vi "acquire sequence to disk.vi"(0 "Image Size":T4={"H Bin"=1, "V Bin"=1, "Left"=1, "Top"=1, "Right"=512, "Bottom"=512} {"Top" min=4 max=2048 step=4; "Left" min=4 max=2048 step=4; "V Bin" min=1 max=2048 step=4; "H Bin" min=1 max=2048 step=4}, 1 "Display?":bool=TRUE, 2 "State In":T5 {"Height" format="%.2f"; "Width" format="%.2f"}, 3 "Frames per acquisition file":u32, 4 "Sequence files handle":T3, 6 "Description Info":string, 7 "Pressing stop automatically runs finish?":bool=TRUE, 9 "Display Window Title":string="Acquired Image", 10 "Operation":enum16{"Start", "Continue", "Finish"}(ring), 11 "Display Window Number":i32, 12 "Number of frames to acquire":i32) -> (15 "Done?":bool, 16 "State Out":T5 {"Height" format="%.2f"; "Width" format="%.2f"}, 18 "Sequence files handle out":T3, 19 "error out":errorcluster)   [LabVIEW 2015]
doc: "Acquires a video sequence into the acquisition RAID directory using the camera handle and buffers already set up (e.g., by ixon acquisition setup.vi). \n\nUse as a sub-vi:\n\nSTARTING: If Start (T)/Continue (F) is True, starts the acquisition from frame 1 and \"State In\" is ignored. If false, continues an earlier acquistision that was temporarily interrupted, using information in \"State In\". \n\nSTOPPING: Program always stops acquisition by calling Camera Stop before it exits. Stop is temporary if Number of frames to acquire is > 0 and the number of frames acquired exceeds that value. In that case, State Out is set so that acquisition can be resumed later. In contrast, if acquisition is stopped by pressing \"Stop\", by an error, or by setting STOP=true as input, the acquisition is over permanently. In that case,the vi writes the header file and frees the acquisition buffers."
uses:
  Glimpse core/Video acquisition state.ctl
  <vilib>/vision/Image Controls.llb/IMAQ Image.ctl
  Glimpse core/Seq file v 1/Offset table.ctl
  Glimpse core/Seq file v 1/Offset.ctl
  Glimpse core/Seq file v 1/file number.ctl
  ixon camera/image size.ctl
  Glimpse core/Sequence files handle.ctt
  h-nu-ixon/Emission filters.ctl
  h-nu-ixon/Laser type.ctt
  ixon1024/HAL camera parameters important.ctt
  ixon1024/ixon readout settings.ctl
  ixon1024/andor acquisition mode.ctl
  Glimpse core/Header2 file data.ctl
  Glimpse core/GLIMPSE Globals.vi
  h-nu-ixon/stage globals.vi
  h-nu shutters/hardware status globals.vi
  fluid handling/Flow cell controller globals.vi
  h-nu-ixon/Microscope ID global.vi
  ixon1024/HAL Camera specifications globals.vi
  Microscope software version global.vi
panel:
  in  "Laser\n(to get strings only)":T1
  in  "Emission filter\n(to get strings only)":T2
  out "Channel switch overhead (ms)":u32
  out "Sequence files directory path":path
  in  "stop":bool
  out "Frame interval (ms)":i16
  out "TTB element zero":u32
  out "Time of 1st frame":dbl
  out "Frames Acquired":u32(slide) scale=0.0..10000.0
  # "Parameters for non-interactive use"
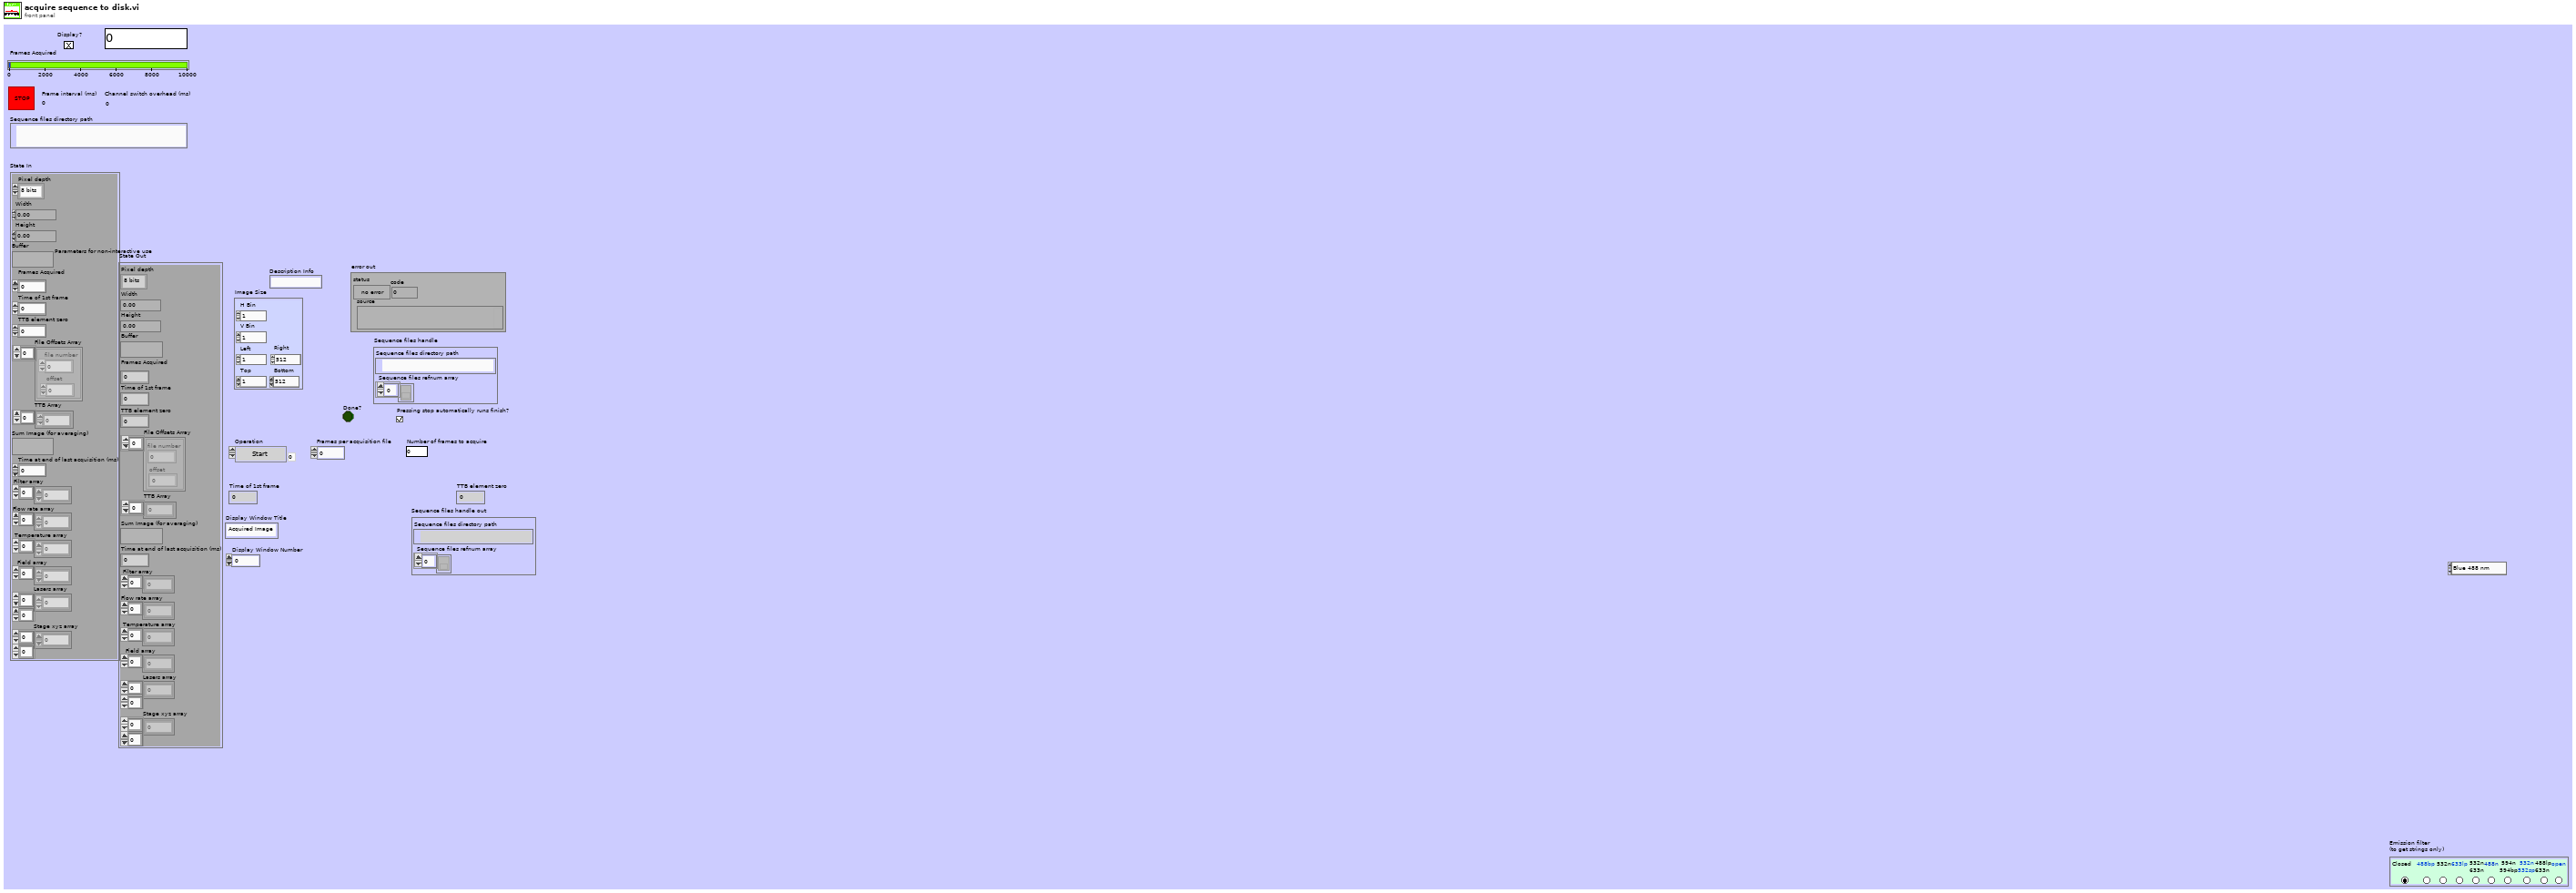
[diagram p1: front panel]
types:
  T1 = typedef "Laser type.ctt" = enum16{"Blue 488 nm", "Green 532 nm", "Orange 594 nm", "Red 633 nm", "IR 780"}
  T2 = typedef "Emission filters.ctl" = enum32{" Closed ", "488bp ", "532n", "633lp ", "532n\n633n", "488n", "594n\n594bp", "532n\n532sp", "488lp\n633n", "open"}
  T3 = typedef "Sequence files handle.ctt" = cluster{"Sequence files directory path":path, "Sequence files refnum array":refnum<file>[]}
  T4 = typedef "image size.ctl" = cluster{"H Bin":i32, "V Bin":i32, "Left":i32, "Top":i32, "Right":i32, "Bottom":i32}
  T5 = typedef "Video acquisition state.ctl" = cluster{"Pixel depth":enum32{"8 bits", "16 bits", "Float", "Complex", "RGB Chunky", "Compressed"}, "Width":dbl, "Height":dbl, "Buffer":T6, "Frames Acquired":u32, "Time of 1st frame":dbl, "TTB element zero":u32, "File Offsets Array":T7, "TTB Array":u32[], "Sum Image (for averaging)":T6, "Time at end of last acquisition (ms)":u32, "Filter array":u16[], "Flow rate array":dbl[], "Temperature array":dbl[], "Field array":u16[], "Lasers array":u16[][], "Stage xyz array":dbl[][]}
  T6 = typedef "IMAQ Image.ctl" = refnum<image>
  T7 = typedef "Offset table.ctl" = cluster{"offset":T8, "file number":T9}[]
  T8 = typedef "Offset.ctl" = i32
  T9 = typedef "file number.ctl" = u8
  T10 = enum32{"8 bits", "16 bits", "Float", "Complex", "RGB Chunky", "Compressed"}
  T11 = typedef "HAL camera parameters important.ctt" = cluster{"Exposure Time (sec)":sgl, "EM CCD Gain":u16, "Readout Settings":T12, "Image Size":cluster{"H Bin":i32, "V Bin":i32, "Left":i32, "Top":i32, "Right":i32, "Bottom":i32}}
  T12 = typedef "ixon readout settings.ctl" = cluster{"Acquisition Mode":T13, "Pixel Rate":enum16{"EM CCD 10 Mhz 14 bits", "EM CCD 5 Mhz 14 bits", "EM CCD 3 Mhz 14 bits", "EM CCD 1 Mhz 16 bits", "Standard CCD 3 Mhz 14 bits", "Standard CCD 1 Mhz 16 bits"}, "High Capacity?":bool, "V Shift Speed (us/row)":enum16{"0.9 (not reccommended)", "1.7  (not reccommended)", "3.3  (not reccommended)", "6.5", "12.9"}, "V Shift Amplitude":enum16{"normal", "+1", "+2", "+3", "+4"}, "Preamp Gain":enum16{"1.0", "2.4", "5.0"}, "Trigger Mode":u32, "Baseline offset":i16, "Baseline clamp":bool}
  T13 = typedef "andor acquisition mode.ctl" = enum16{"(do not use)", "Single Scan", "Accumulate", "Kinetics", "Fast Kinetics", "Kinetics Run till Abort", "Frame Transfer", "Frame Transfer Run till Abort", "(do not use) ", "Time Delayed Integration"}
  T14 = typedef "shutters status.ctl" = cluster{"Laser":T1, "Status":bool}[]
  T15 = typedef "Header2 file data.ctl" = cluster{"Camera":string, "Microscope":string, "Microscope software version":string, "Laser names":string[], "Filter names":string[], "Lasers array":u16[][], "Filter array":u16[], "Flow rate array":dbl[], "Temperature array":dbl[], "Field array":u16[], "Is header2 info present?":bool, "Description Info":string, "Stage xyz array":dbl[][]}
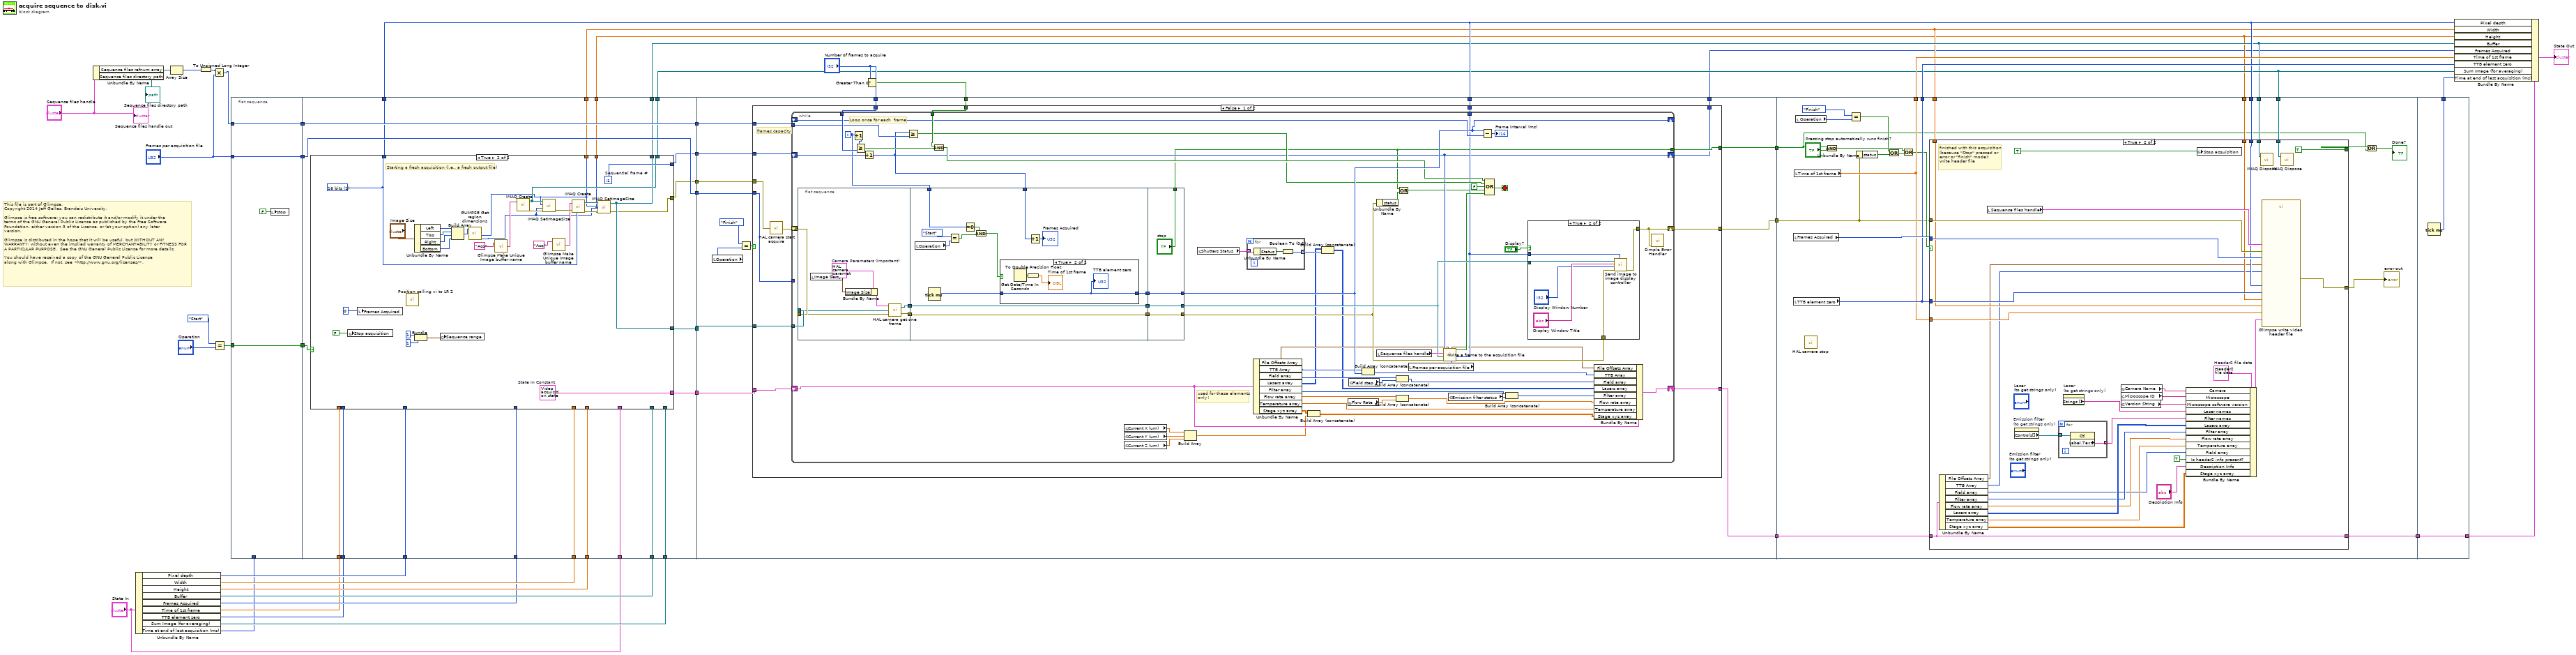
[diagram p0: block diagram]
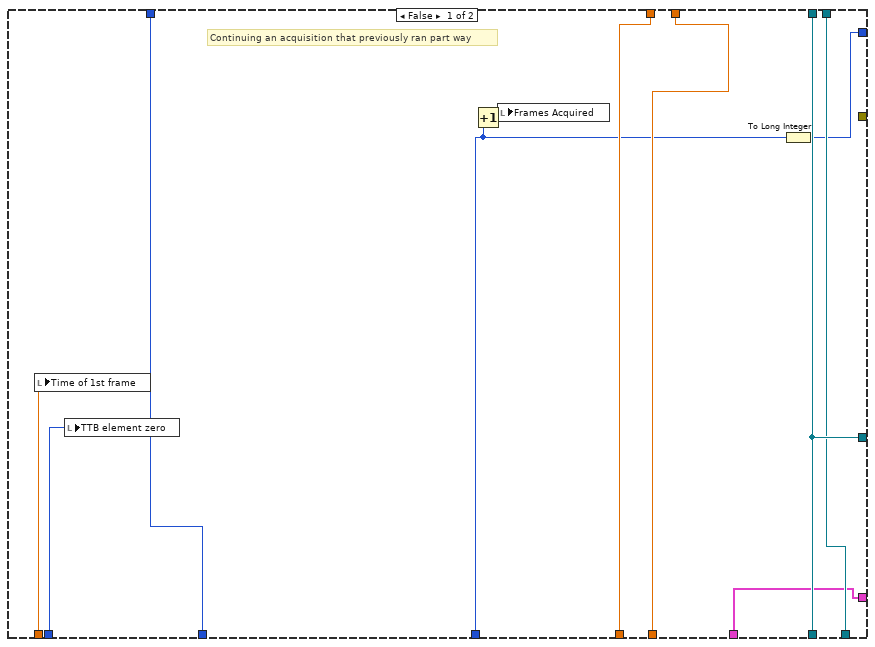
[diagram p2: hidden frame]
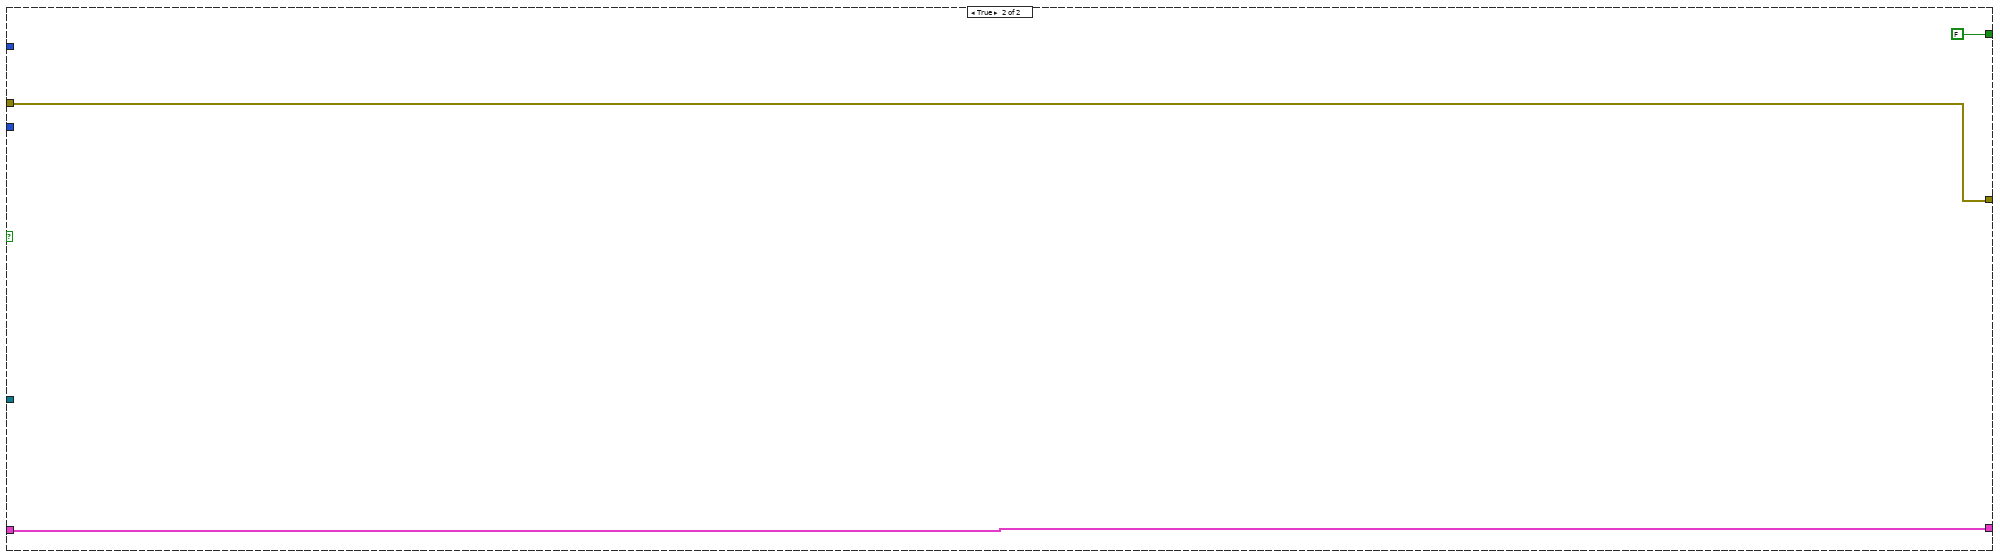
[diagram p5: hidden frame]
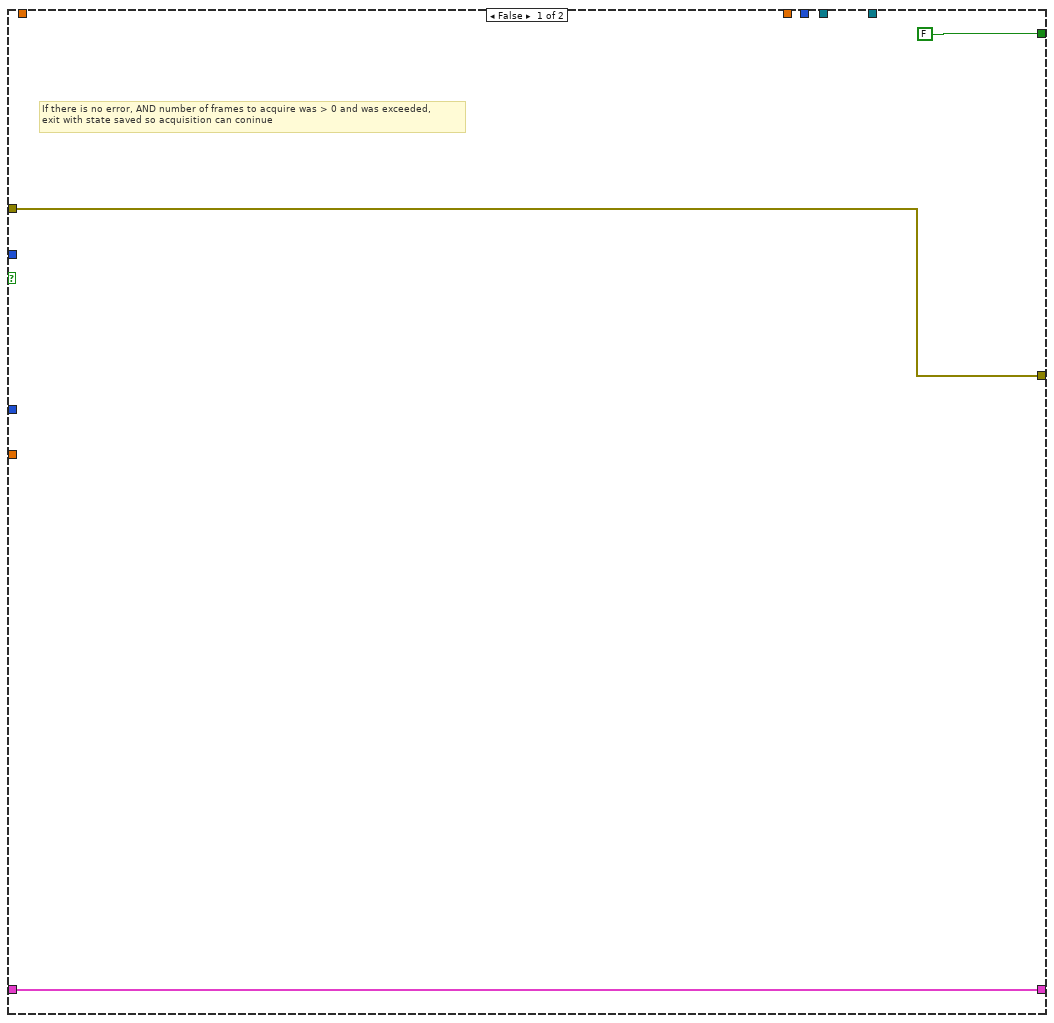
[diagram p6: hidden frame]
diagram:
  # "This file is part of Glimpse. \nCopyright 2014 Jeff Gelles, Brandeis University.    \n\nGlimpse is free software: you can redistribute it and/or modify it under the \nterms of the GNU General Public License as published by the Free Software \nFoundation, either version 3 of the License, or (at your option) any later \nversion.\n\nGlimpse is distributed in the hope that it will be useful, but WITHOUT ANY \nWARRANTY; without even the implied warranty of MERCHANTABILITY or FITNESS FOR \nA PARTICULAR PURPOSE.  See the GNU General Public License for more details.\n\nYou should have received a copy of the GNU General Public License\nalong with Glimpse.  If not, see <http://www.gnu.org/licenses/>."
  n1 = Unbundle By Name("Sequence files handle") -> ("Sequence files refnum array"=w9:refnum<file>[], "Sequence files directory path"=→"Sequence files directory path":path)
  n2 = Unbundle By Name("State In") -> ("Pixel depth"=w36:T10, "Width"=w35:dbl, "Height"=w34:dbl, "Buffer"=w33:T6, "Frames Acquired"=w32:u32, "Time of 1st frame"=w30:dbl, "TTB element zero"=w29:u32, "Sum Image (for averaging)"=w25:T6, "Time at end of last acquisition (ms)"=w6:u32)
  n3 = Array Size(array=w9) -> (size(s)=w26:i32)
  n4 = To Unsigned Long Integer(number=w26) -> (unsigned 32bit integer=w45:u32)
  n5 = Multiply(x=w45, y="Frames per acquisition file") -> (x*y=w46:u32)
  n6 = Equal?(x=enum16{"Start", "Continue", "Finish"}."Start", y="Operation") -> (x = y?=w19:bool)
  n7 = flat-sequence {
    tunnel: w19 -> [w51]
    tunnel: "Frames per acquisition file" -> [w52]
    tunnel: w46 -> [w53]
    tunnel: [w53] -> w13
    tunnel: [w52] -> w12
    tunnel: [w51] -> w11
    tunnel: w6 -> [w47]
    tunnel: [w73] -> w41
    tunnel: [w72] -> w40
    tunnel: [w71] -> w39
    tunnel: [w70] -> w38
    tunnel: [w69] -> w22
    tunnel: [w68] -> w16
    tunnel: [w67] -> w15
    tunnel: [w66] -> w20
    tunnel: w36 -> [w65]
    tunnel: w35 -> [w64]
    tunnel: w34 -> [w56]
    tunnel: w33 -> [w63]
    tunnel: w32 -> [w62]
    tunnel: [w61] -> w31
    tunnel: w30 -> [w60]
    tunnel: w29 -> [w59]
    tunnel: w25 -> [w58]
    tunnel: [w57] -> w21
    tunnel: w13 -> [w73]
    tunnel: w12 -> [w72]
    tunnel: w11 -> [w74]
    tunnel: "State In" -> [w55]
    tunnel: [w54] -> w4
    tunnel: w41 -> [w128]
    tunnel: w40 -> [w127]
    tunnel: [w122] -> w42
    tunnel: w39 -> [w116]
    tunnel: w38 -> [w126]
    tunnel: w31 -> [w125]
    tunnel: "Number of frames to acquire" -> [w124]
    tunnel: w23 -> [w123]
    tunnel: w22 -> [w121]
    tunnel: [w120] -> w17
    tunnel: [w115] -> w14
    tunnel: w4 -> [w114]
    tunnel: [w113] -> w3
    tunnel: w42 -> [w245]
    tunnel: [w264] -> w28
    tunnel: [w263] -> w27
    tunnel: w15 -> [w262]
    tunnel: w16 -> [w261]
    tunnel: w22 -> [w260]
    tunnel: w21 -> [w257]
    tunnel: w20 -> [w256]
    tunnel: w17 -> [w246]
    tunnel: w3 -> [w244]
    tunnel: [w243] -> w2
    tunnel: [w304] -> w7
    tunnel: [w303] -> w1
    tunnel: w2 -> [w303]
    frame #0 {
      n8 = Tick Count (ms)() -> (millisecond timer value=w48:u32)
      n9 = Subtract(x=w48, y=w47) -> (x-y=→"Channel switch overhead (ms)":u32)
      n10 = local write "stop"(FALSE ("stop")) -> ()
    }
    frame #1 {
      n11 = case shown="True" w74 {
        tunnel: [_ w101] -> w71
        tunnel: [w77 w105] -> w70
        tunnel: [w81 w95] -> w69
        tunnel: [w85 w88] -> w68
        tunnel: [w84 w87] -> w67
        tunnel: [w82 w104] -> w66
        tunnel: w65 -> [w81 _]
        tunnel: w64 -> [w85 _]
        tunnel: w56 -> [w84 _]
        tunnel: w63 -> [w82 _]
        tunnel: w62 -> [w83 _]
        tunnel: [w82 w104] -> w61
        tunnel: w60 -> [w80 _]
        tunnel: w59 -> [w79 _]
        tunnel: w58 -> [w78 _]
        tunnel: [w78 w96] -> w57
        tunnel: [w75 w86] -> w54
        tunnel: w55 -> [w75 _]
        frame False {
          # "Continuing an acquisition that previously ran part way"
          n12 = local write "Time of 1st frame"(w80) -> ()
          n13 = local write "TTB element zero"(w79) -> ()
          n14 = Increment(x=w83) -> (x+1=w76:u32)
          n15 = local write "Frames Acquired"(w76) -> ()
          n16 = To Long Integer(number=w83) -> (32bit integer=w77:i32)
        }
        frame True {
          w86 = T5 {"Pixel depth"=enum."8 bits", "Width"=0.0, "Height"=0.0, "Buffer"=refnum, "Frames Acquired"=0, "Time of 1st frame"=0.0, "TTB element zero"=0, "File Offsets Array"=[], "TTB Array"=[], "Sum Image (for averaging)"=refnum, "Time at end of last acquisition (ms)"=0, "Filter array"=[], "Flow rate array"=[], "Temperature array"=[], "Field array"=[], "Lasers array"=[], "Stage xyz array"=[]}  # State In Constant
          w95 = u32 1 items=["8 bits", "16 bits", "Float", "Complex", "RGB", "HSL"] ("Image Type")
          w105 = -1  # Sequential frame #
          # "Starting a fresh acquisition (i.e., a fresh output file)"
          n17 = global write "GLIMPSE Globals.vi" "Stop acquisition"(FALSE ("Stop acquisition")) -> ()
          n18 = local write "Frames Acquired"(u32 0 ("Frames Acquired")) -> ()
          n19 = call "Position calling vi to LR 2.vi"() -> ()  [unwired: 2 in, 4 out]
          n20 = Unbundle By Name("Image Size") -> ("Left"=w94:i32, "Top"=w93:i32, "Right"=w92:i32, "Bottom"=w91:i32)
          n21 = Bundle(i16 1, i16 1) -> (w108:cluster{i16, i16})  [unwired: 1 out]
          n22 = global write "GLIMPSE Globals.vi" "Sequence range"(w108) -> ()
          n23 = Build Array(w94, w93, w92, w91) -> (w89:i32[])
          n24 = call "GLIMPSE Get region dimensions.vi"("x1y1x2y2"=w89) -> ("y size"=w87:u16, "x size"=w88:u16)  [unwired: 9 out]
          n25 = call "Glimpse Make Unique Image buffer name.vi"("Buffer  base name"="Acq" ("Image Name")) -> ("Image Name"=w99:string)  [unwired: 1 out]
          n26 = call "IMAQ Create"("Image Name"=w99) -> ("New Image"=w96:T6, "error out"=w103:errorcluster)  [unwired: 3 in, 1 out]
          n27 = call "IMAQ SetImageSize"("error in (no error)"=w103, "Y Resolution"=w87, "X Resolution"=w88, "Image"=w96) -> ("error out"=w102:errorcluster)  [unwired: 2 out]
          n28 = call "Glimpse Make Unique Image buffer name.vi"("Buffer  base name"="Acq" ("Image Name")) -> ("Image Name"=w97:string)  [unwired: 1 out]
          n29 = call "IMAQ Create"("Image Name"=w97, "Image Type"=w95, "error in (no error)"=w102) -> ("New Image"=w107:T6, "error out"=w106:errorcluster)  [unwired: 1 in, 1 out]
          n30 = call "IMAQ SetImageSize"("error in (no error)"=w106, "Y Resolution"=w87, "X Resolution"=w88, "Image"=w107) -> ("error out"=w101:errorcluster, "Image Out"=w104:T6)  [unwired: 1 out]
        }
      }
    }
    frame #2 {
      n31 = local read "Operation"() -> (w118:enum16{"Start", "Continue", "Finish"})
      n32 = Equal?(x=enum16{"Start", "Continue", "Finish"}."Finish", y=w118) -> (x = y?=w117:bool)
      n33 = case shown="False" w117 {
        tunnel: w128 -> [w142 _]
        tunnel: w127 -> [w141 _]
        tunnel: w116 -> [w134 w241]
        tunnel: w126 -> [w140 _]
        tunnel: w125 -> [w139 _]
        tunnel: w124 -> [w138 _]
        tunnel: w123 -> [w137 _]
        tunnel: [w136 w241] -> w122
        tunnel: w121 -> [w135 _]
        tunnel: [w132 FALSE] -> w120
        tunnel: [w131 _] -> w115
        tunnel: w114 -> [w130 w240]
        tunnel: [w129 w240] -> w113
        frame False {
          # "frames capacity"
          n34 = call "HAL camera start acquire.vi"("error in"=w134) -> ("error out"=w133:errorcluster)
          n35 = while {
            tunnel: w142 -> [w199]
            tunnel: w141 -> [_]
            tunnel: w139 -> [w191]
            tunnel: w138 -> [w202]
            tunnel: w137 -> [w201]
            shift-right: [w176] -> w131
            shift-left: w140 -> [w195]
            shift-right: [w177] -> w136
            shift-left: w133 -> [w190]
            tunnel: w135 -> [w178]
            shift-right: [w186] -> _
            shift-left: _ -> [w192]
            tunnel: [w169] -> w132
            shift-right: [w165] -> w129
            shift-left: w130 -> [w166]
            i -> [w187]
            stop <- w183 stop-if-true
            # "used for these elements\nonly!"
            # "Loop once for each  frame"
            n36 = flat-sequence {
              tunnel: w191 -> [w212]
              tunnel: w190 -> [w211]
              tunnel: [w210] -> w185
              tunnel: [w209] -> w184
              tunnel: w184 -> [w224]
              tunnel: w185 -> [w223]
              tunnel: w187 -> [w221]
              tunnel: w176 -> [w213]
              tunnel: [w224] -> w172
              tunnel: [w223] -> w171
              tunnel: [w220] -> w170
              tunnel: [w230] -> w186
              tunnel: [w231] -> w189
              tunnel: [w232] -> w173
              tunnel: w172 -> [w232]
              tunnel: w171 -> [w231]
              tunnel: w170 -> [w230]
              tunnel: ["stop"] -> w169
              frame #0 {
                w207 = T11 {"Exposure Time (sec)"=0.0, "EM CCD Gain"=0, "Readout Settings"={"Acquisition Mode"=enum."(do not use)", "Pixel Rate"=enum."EM CCD 10 Mhz 14 bits", "High Capacity?"=FALSE, "V Shift Speed (us/row)"=enum."0.9 (not reccommended)", "V Shift Amplitude"=enum."normal", "Preamp Gain"=enum."1.0", "Trigger Mode"=0, "Baseline offset"=0, "Baseline clamp"=FALSE}, "Image Size"={"H Bin"=0, "V Bin"=0, "Left"=0, "Top"=0, "Right"=0, "Bottom"=0}}  # Camera Parameters (important)
                n37 = local read "Image Size"() -> (w206:T4)
                n38 = Bundle By Name(cluster=w207, "Image Size"=w206) -> (w208:T11)
                n39 = call "HAL camera get one frame.vi"("error in"=w211, "New Image"=w212, "Camera Parameters (important)"=w208) -> ("error out"=w209:errorcluster, "Image Out"=w210:T6)
              }
              frame #1 {
                n40 = local read "Operation"() -> (w218:enum16{"Start", "Continue", "Finish"})
                n41 = Tick Count (ms)() -> (millisecond timer value=w222:u32)
                n42 = Equal?(x=enum16{"Start", "Continue", "Finish"}."Start", y=w218) -> (x = y?=w216:bool)
                n43 = Equal To 0?(x=w221) -> (x = 0?=w217:bool)
                n44 = And(x=w217, y=w216) -> (x .and. y?=w215:bool)
                n45 = case shown="True" w215 {
                  tunnel: [w225 w226] -> w220
                  tunnel: w222 -> [w225 w226]
                  frame False {
                  }
                  frame True {
                    n46 = Get Date/Time In Seconds() -> (seconds since 1Jan1904=w228:timestamp)
                    n47 = To Double Precision Float(number=w228) -> (double precision float=→"Time of 1st frame":dbl)
                    "TTB element zero" <- w226
                  }
                }
                n48 = Increment(x=w213) -> (x+1=→"Frames Acquired":i32)
              }
              frame #2 {
              }
            }
            n49 = Increment(x=w187) -> (x+1=w193:i32)
            n50 = Greater Or Equal?(x=w193, y=w202) -> (x >= y?=w200:bool)
            n51 = Increment(x=w195) -> (x+1=w176:i32)
            n52 = Greater Or Equal?(x=w176, y=w199) -> (x >= y?=w180:bool)
            n53 = And(x=w201, y=w200) -> (x .and. y?=w181:bool)
            n54 = global read "stage globals.vi" "Current X (um)"() -> (w149:ext)
            n55 = global read "stage globals.vi" "Current Y (um)"() -> (w148:ext)
            n56 = global read "stage globals.vi" "Current Z (um)"() -> (w147:ext)
            n57 = Build Array(w149, w148, w147) -> (w144:ext[])
            n58 = global read "hardware status globals.vi" "Shutters Status"() -> (w155:T14)
            n59 = for {
              tunnel: w155 -> [w205] mode=indexing
              tunnel: [w203] -> w154 mode=indexing
              n60 = Unbundle By Name(w205) -> ("Status"=w204:bool)
              n61 = Boolean To (0,1)(Boolean=w204) -> (0, 1=w203:i16)
            }
            n62 = Unbundle By Name(w166) -> ("File Offsets Array"=w168:T7, "TTB Array"=w167:u32[], "Field array"=w162:u16[], "Lasers array"=w153:u16[][], "Filter array"=w158:u16[], "Flow rate array"=w156:dbl[], "Temperature array"=w146:dbl[], "Stage xyz array"=w145:dbl[][])
            n63 = Build Array (concatenate)(w145, w144) -> (w143:ext[][])
            n64 = Build Array (concatenate)(w153, w154) -> (w152:u16[][])
            n65 = global read "Flow cell controller globals.vi" "Flow Rate"() -> (w150:dbl)
            n66 = global read "stage globals.vi" "Field step"() -> (w160:i16)
            n67 = Build Array (concatenate)(w167, w186) -> (w163:u32[])
            n68 = Unbundle By Name(w173) -> ("status"=w175:bool)
            n69 = local read "Sequence files handle"() -> (w197:T3)
            n70 = Build Array (concatenate)(w162, w160) -> (w161:u16[])
            n71 = Build Array (concatenate)(w156, w150) -> (w151:dbl[])
            n72 = Or(x=w169, y=w175) -> (x .or. y?=w174:bool)
            n73 = local read "Frames per acquisition file"() -> (w198:u32)
            n74 = call "Write a frame to the acquisition file.vi"("Pixel depth"=w178, "Frames per acquisition file"=w198, "Offset table in"=w168, "error in"=w173, "Image In"=w189, "Sequence files handle"=w197, "Last frame number written in"=w176) -> ("error out"=w188:errorcluster, "Stop"=w182:bool, "Offset table out"=w164:T7)  [unwired: 1 in, 1 out]
            n75 = global read "hardware status globals.vi" "Emission filter status"() -> (w159:T2)
            n76 = Subtract(x=w186, y=w192) -> (x-y=→"Frame interval (ms)":u32)
            n77 = Compound Arithmetic op=OR(w181, w180, FALSE ("value"), w174, w182) -> (w183:bool)
            n78 = Build Array (concatenate)(w158, w159) -> (w157:u32[])
            n79 = case shown="True" "Display?" {
              tunnel: w189 -> [_ w238]
              tunnel: w188 -> [w233 w235]
              tunnel: [w233 w234] -> w177
              tunnel: w178 -> [_ w239]
              frame False {
              }
              frame True {
                n80 = call "Send image to image display controller.vi"("Image"=w238, "Window Title"="Display Window Title", "Window Number"="Display Window Number", "error in"=w235, "Image Type"=w239) -> ("error out"=w234:errorcluster)  [unwired: 2 in, 3 out]
              }
            }
            n81 = Bundle By Name(cluster=w166, "File Offsets Array"=w164, "TTB Array"=w163, "Field array"=w161, "Lasers array"=w152, "Filter array"=w157, "Flow rate array"=w151, "Temperature array"=w146, "Stage xyz array"=w143) -> (w165:T5)
            n82 = call <vilib>:"Simple Error Handler.vi"("error in (no error)"=w177) -> ()  [unwired: 1 in, 8 out]
          }
        }
        frame True {
        }
      }
    }
    frame #3 {
      n83 = local read "Frames Acquired"() -> (w265:u32)
      n84 = local read "TTB element zero"() -> (w264:u32)
      n85 = local read "Time of 1st frame"() -> (w263:dbl)
      n86 = local read "Operation"() -> (w250:enum16{"Start", "Continue", "Finish"})
      n87 = call "HAL camera stop.vi"() -> ()  [unwired: 1 in]
      n88 = And(x=w246, y="Pressing stop automatically runs finish?") -> (x .and. y?=w249:bool)
      n89 = Equal?(x=enum16{"Start", "Continue", "Finish"}."Finish", y=w250) -> (x = y?=w251:bool)
      n90 = Unbundle By Name(w245) -> ("status"=w254:bool)
      n91 = Or(x=w251, y=w254) -> (x .or. y?=w255:bool)
      n92 = Or(x=w249, y=w255) -> (x .or. y?=w253:bool)
      n93 = case shown="True" w253 {
        tunnel: [w268 w299] -> w259
        tunnel: w245 -> [w268 w297]
        tunnel: w265 -> [_ w296]
        tunnel: w264 -> [_ w295]
        tunnel: w263 -> [_ w294]
        tunnel: w262 -> [_ w293]
        tunnel: w261 -> [_ w292]
        tunnel: w260 -> [_ w291]
        tunnel: [FALSE ("Stop acquisition") TRUE ("Stop acquisition")] -> w258
        tunnel: w257 -> [_ w289]
        tunnel: w256 -> [_ w288]
        tunnel: w244 -> [w266 w287]
        tunnel: [w266 w287] -> w243
        frame False {
          # "If there is no error, AND number of frames to acquire was > 0 and was exceeded,\nexit with state saved so acquisition can coninue"
        }
        frame True {
          w277 = T15 {"Camera"="", "Microscope"="", "Microscope software version"="", "Laser names"=[], "Filter names"=[], "Lasers array"=[], "Filter array"=[], "Flow rate array"=[], "Temperature array"=[], "Field array"=[], "Is header2 info present?"=FALSE, "Description Info"="", "Stage xyz array"=[]}  # Header2 file data
          # "finished with this acquisition\n(because \"Stop\" pressed or\nerror or \"finish\" mode); \nwrite header file"
          n94 = Unbundle By Name(w287) -> ("File Offsets Array"=w286:T7, "TTB Array"=w285:u32[], "Field array"=w272:u16[], "Filter array"=w275:u16[], "Flow rate array"=w274:dbl[], "Lasers array"=w276:u16[][], "Temperature array"=w273:dbl[], "Stage xyz array"=w269:dbl[][])
          n95 = local read "Sequence files handle"() -> (w298:T3)
          n96 = property on="Emission filter\n(to get strings only)" class="RadioBtnsControl (strict)"() -> ("Controls[]"=w281:refnum<vi>[])  [unwired: 2 in, 2 out]
          n97 = for {
            tunnel: w281 -> [w302] mode=indexing
            tunnel: [w301] -> w283 mode=indexing
            n98 = property class="Ctl"(reference=w302) -> ("Label.Text"=w301:string)  [unwired: 1 in, 2 out]
          }
          n99 = property on="Laser\n(to get strings only)" class="Enum (strict)"() -> ("Strings []"=w282:string[])  [unwired: 2 in, 2 out]
          n100 = global read "HAL Camera specifications globals.vi" "Camera Name"() -> (w278:string)
          n101 = global read "Microscope ID global.vi" "Microscope ID"() -> (w279:string)
          n102 = global read "Microscope software version global.vi" "Version String"() -> (w280:string)
          n103 = Bundle By Name(cluster=w277, "Camera"=w278, "Microscope"=w279, "Microscope software version"=w280, "Laser names"=w282, "Filter names"=w283, "Lasers array"=w276, "Filter array"=w275, "Flow rate array"=w274, "Temperature array"=w273, "Field array"=w272, "Is header2 info present?"=TRUE, "Description Info"="Description Info", "Stage xyz array"=w269) -> (w271:T15)
          n104 = global write "GLIMPSE Globals.vi" "Stop acquisition"(TRUE ("Stop acquisition")) -> ()
          n105 = call "IMAQ Dispose"("Image"=w288) -> ()  [unwired: 2 in, 4 out]
          n106 = call "Glimpse write video header file.vi"("Number of frames"=w296, "Sequence files handle"=w298, "Pixel depth\n(0=8 bit; 1= 16 bit)"=w291, "error in"=w297, "TTB Array"=w285, "Offsets Array"=w286, "Header2 file data"=w271, "Region width"=w292, "Region height"=w293, "Element 0 of TTB"=w295, "time of 1st frame, \nsec since 1/1/04"=w294) -> ("error out"=w299:errorcluster)  [unwired: 8 in]
          n107 = call "IMAQ Dispose"("Image"=w289) -> ()  [unwired: 2 in, 4 out]
        }
      }
      "error out" <- w259
      n108 = Or(x=w258, y=w246) -> (x .or. y?=→"Done?":bool)
      n109 = call <vilib>:"General Error Handler.vi"() -> ()  [unwired: 3 in, 13 out]
    }
    frame #4 {
      n110 = Tick Count (ms)() -> (millisecond timer value=w304:u32)
    }
  }
  n111 = Greater Than 0?(x="Number of frames to acquire") -> (x > 0?=w23:bool)
  n112 = Bundle By Name(cluster=w1, "Pixel depth"=w22, "Width"=w16, "Height"=w15, "Buffer"=w20, "Frames Acquired"=w14, "Time of 1st frame"=w27, "TTB element zero"=w28, "Sum Image (for averaging)"=w21, "Time at end of last acquisition (ms)"=w7) -> (→"State Out":T5)
  "Sequence files handle out" <- "Sequence files handle"
